vi "Fill W.vi"(7 "i":i32, 10 "W In":u32[](array[numeric]), 11 "Chunk":u32[](array[numeric])) -> (2 "W":u32[](array[numeric]), 5 "W[i]":u32)   [LabVIEW 2018, in "Crypto.lvlib" / "SHA-256.lvclass"]
uses:
  SHA-256.lvclass
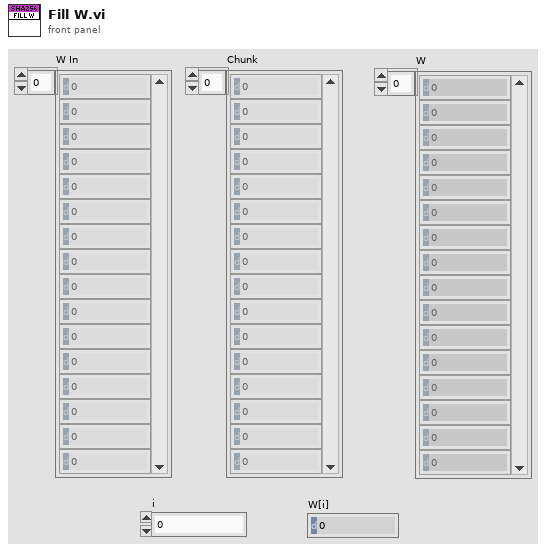
[diagram p1: front panel]
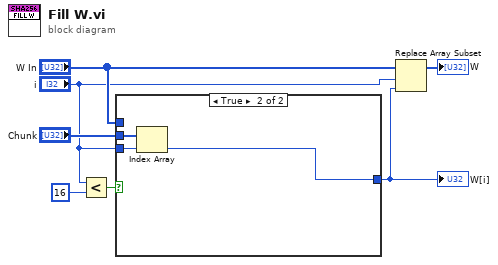
[diagram p0: block diagram]
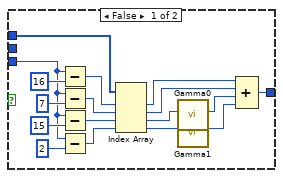
[diagram p2: hidden frame]
diagram:
  n1 = Less?(x="i", y=16) -> (x < y?=w3:bool)
  n2 = case shown="True" w3 {
    tunnel: "W In" -> [w14 _]
    tunnel: [w13 w26] -> w5
    tunnel: "Chunk" -> [_ w27]
    tunnel: "i" -> [w12 w25]
    frame False {
      n3 = Subtract(x=w12, y=16) -> (x-y=w17:i32)
      n4 = Subtract(x=w12, y=7) -> (x-y=w18:i32)
      n5 = Subtract(x=w12, y=15) -> (x-y=w24:i32)
      n6 = Subtract(x=w12, y=2) -> (x-y=w21:i32)
      n7 = Index Array(array=w14, index #1=w17, index #2=w18, index #3=w24, index #4=w21) -> (element #1=w16:u32, element #2=w15:u32, element #3=w11:u32, element #4=w9:u32)
      n8 = call "Gamma0.vi"("Value"=w11) -> ("Gamma 0"=w10:u32)  [unwired: 10 in]
      n9 = call "Gamma1.vi"("Value"=w9) -> ("Gamma 1"=w8:u32)  [unwired: 10 in]
      n10 = Compound Arithmetic op=ADD(w16, w15, w10, w8) -> (w13:u32)
    }
    frame True {
      n11 = Index Array(array=w27, index=w25) -> (element=w26:u32)
    }
  }
  "W[i]" <- w5
  n12 = Replace Array Subset(array="W In", new element=w5, index="i") -> (→"W":u32[])
